vi "b.vi"(8 "error in (no error)":errorcluster, 11 "OK&NG":refnum<vi>) -> (0 "error out":errorcluster, 3 "OK NG out":refnum<vi>)   [LabVIEW 2013]
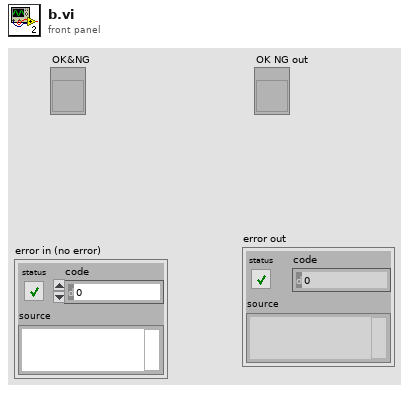
[diagram p1: front panel]
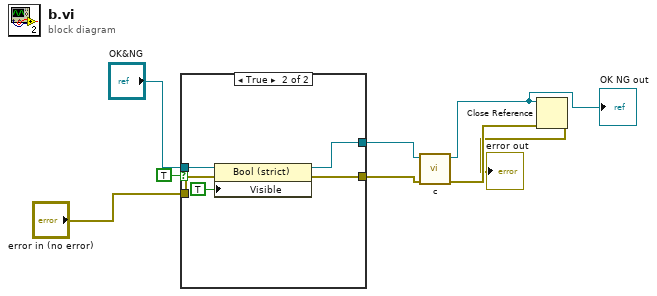
[diagram p0: block diagram]
diagram:
  n1 = case shown="True" TRUE {
    tunnel: "OK&NG" -> [w10 w15]
    tunnel: "error in (no error)" -> [w9 w13]
    tunnel: [w10 w12] -> w6
    tunnel: [w9 w11] -> w5
    frame False {
    }
    frame True {
      n2 = property class="Bool (strict)"(reference=w15, error in=w13, "Visible"=TRUE) -> (reference out=w12:refnum<vi>, error out=w11:errorcluster)
    }
  }
  n3 = call "c.vi"("error in (no error)"=w5, "OK&NG"=w6) -> ("error out"=w4:errorcluster, "OK NG out"=w2:refnum<vi>)  [unwired: 8 in]
  "OK NG out" <- w2
  n4 = Close Reference(reference=w2, error in (no error)=w4) -> (error out=→"error out":errorcluster)
